vi "MOTOR Configure Speed.vi"(8 "error in (no error)":errorcluster, 10 "Message Data":variant, 11 "Data Cluster in":T1={"Tango HW"={"VISA resource"="", "Baud Rate (115200)"=2, "lAnInterfaceType"=0, "bAShowProt"=15}, "Writer Queue"=refnum, "Status"=FALSE, "Abs Position"=[], "Axis Velocity"={"dX"=0.0, "dY"=0.0, "dZ"=0.0, "dA"=0.0}, "acceleration "=0.0, "Z direction"=enum."Up", "Position Mode"="", "plLSID"=0}) -> (0 "error out":errorcluster, 3 "Data Cluster out":T1={"Tango HW"={"VISA resource"="", "Baud Rate (115200)"=2, "lAnInterfaceType"=0, "bAShowProt"=15}, "Writer Queue"=refnum, "Status"=FALSE, "Abs Position"=[], "Axis Velocity"={"dX"=0.0, "dY"=0.0, "dZ"=0.0, "dA"=0.0}, "acceleration "=0.0, "Z direction"=enum."Up", "Position Mode"="", "plLSID"=0})   [LabVIEW 2020, in "MOTOR.lvlib"]
uses:
  MOTOR.lvlib
  PS Hardware Configuration.ctl
  support/Message Queue/Message Cluster.ctl
  support/HW Message Cluster.ctl
  support/PCT FGV CMD.ctl
  support/Message Queue/Message Queue.lvlib
  <instrlib>/Tango_DLL/Tango_DLL.lvlib
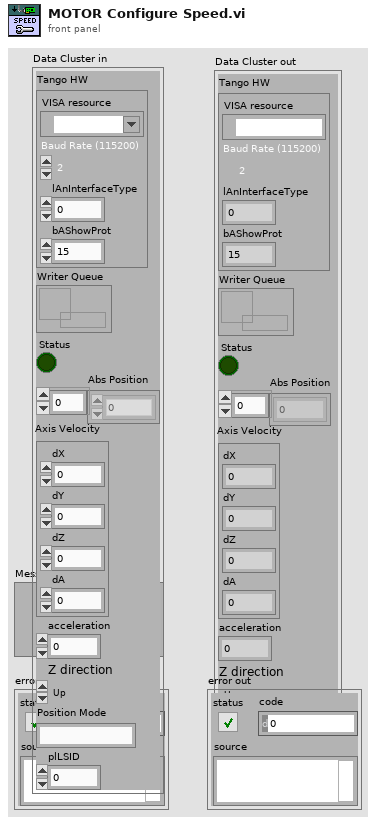
[diagram p1: front panel]
types:
  T1 = typedef "MOTOR.lvlib/PS Hardware Configuration.ctl" = cluster{"Tango HW":cluster{"VISA resource":refnum<visa-resource-name>, "Baud Rate (115200)":i32, "lAnInterfaceType":i32, "bAShowProt":i32}, "Writer Queue":refnum<queue>, "Status":bool, "Abs Position":i32[], "Axis Velocity":cluster{"dX":dbl, "dY":dbl, "dZ":dbl, "dA":dbl}, "acceleration ":dbl, "Z direction":enum16{"Up", "Down"}, "Position Mode":string, "plLSID":i32}
  T2 = typedef "PCT FGV CMD.ctl" = enum16{"INIT", "GET", "SET"}
  T3 = typedef "Message Queue.lvlib/HW Message Cluster.ctl" = cluster{"Writer Queue":refnum<queue>, "Writer Data":T4}
  T4 = typedef "Message Queue.lvlib/Message Cluster.ctl" = cluster{"Message":string, "Message Data":variant}
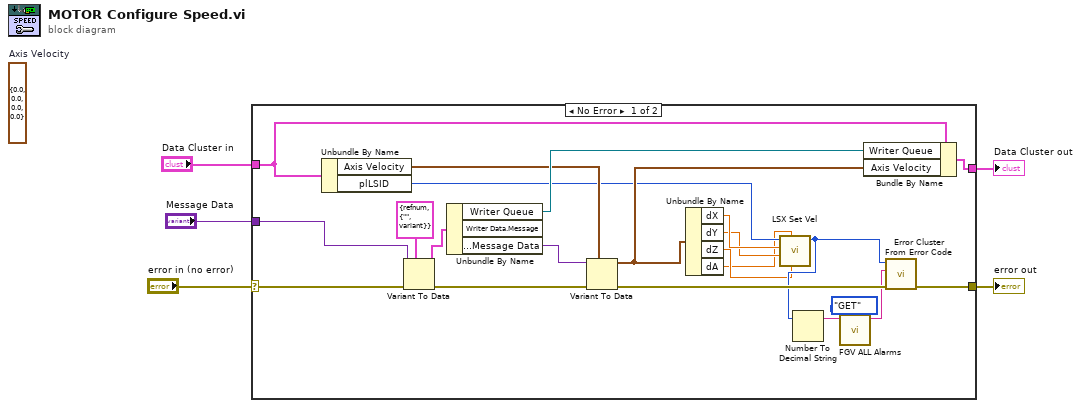
[diagram p0: block diagram]
diagram:
  (unwired) cluster{"dX":dbl, "dY":dbl, "dZ":dbl, "dA":dbl} {"dX"=0.0, "dY"=0.0, "dZ"=0.0, "dA"=0.0}  # Axis Velocity
  n1 = case shown="No Error" "error in (no error)" {
    selector: "error in (no error)" -> [w20 w28]
    tunnel: "Message Data" -> [w19 _]
    tunnel: [w18 w29] -> w4
    tunnel: "Data Cluster in" -> [w21 w29]
    tunnel: [w15 w28] -> w2
    frame No Error {
      n2 = Unbundle By Name(w21) -> ("Axis Velocity"=w17:cluster{"dX":dbl, "dY":dbl, "dZ":dbl, "dA":dbl}, "plLSID"=w11:i32)
      n3 = Variant To Data(error in=w20, type=T3 {"Writer Queue"=refnum, "Writer Data"={"Message"="", "Message Data"=variant}}, Variant=w19) -> (data=w27:T3, error out=w25:errorcluster)
      n4 = Unbundle By Name(w27) -> ("Writer Queue"=w24:refnum<queue>, "Writer Data.Message Data"=w26:variant)  [unwired: 1 out]
      n5 = Variant To Data(error in=w25, type=w17, Variant=w26) -> (data=w16:cluster{"dX":dbl, "dY":dbl, "dZ":dbl, "dA":dbl}, error out=w22:errorcluster)
      n6 = Unbundle By Name(w16) -> ("dX"=w9:dbl, "dY"=w8:dbl, "dZ"=w7:dbl, "dA"=w6:dbl)
      n7 = call <instrlib>:"LSX Set Vel.vi"("dA"=w7, "dZ"=w6, "dY"=w8, "dX"=w9, "lLSID"=w11) -> ("function return"=w10:i32)  [unwired: 5 in, 1 out]
      n8 = Number To Decimal String(number=w10) -> (decimal integer string=w13:string)  [unwired: 1 in]
      n9 = call "FGV ALL Alarms.vi"("CMD"=PCT_FGV_CMD."GET", "name"=w13) -> ("Alarm MSG out"=w12:string)  [unwired: 8 in, 1 out]
      n10 = Bundle By Name(cluster=w21, "Writer Queue"=w24, "Axis Velocity"=w16) -> (w18:T1)
      n11 = call <vilib>:"Error Cluster From Error Code.vi"("error in (no error)"=w22, "error message (\"\")"=w12, "error code (0)"=w10) -> ("error out"=w15:errorcluster)  [unwired: 6 in]
    }
    frame Error {
    }
  }
  "Data Cluster out" <- w4
  "error out" <- w2
